vi "SpectralCoclustering.vi"(8 "error in":errorcluster) -> (0 "error out":errorcluster, 3 "out":refnum<class "SpectralCoclustering.lvclass">)   [LabVIEW 2020]
doc: "Spectral Co-Clustering algorithm (Dhillon, 2001).\n\n Clusters rows and columns of an array `X` to solve the relaxed\n normalized cut of the bipartite graph created from `X` as follows:\n the edge between row vertex `i` and column vertex `j` has weight\n `X[i, j]`.\n\n The resulting bicluster structure is block-diagonal, since each\n row and each column belongs to exactly one bicluster.\n\n Supports sparse matrices, as long as they are nonnegative.\n\n Read more in the :ref:`User Guide <spectral_coclustering>`.\n\n Parameters\n ----------\n n_clusters : int, default=3\n The number of biclusters to find.\n\n svd_method : {'randomized', 'arpack'}, default='randomized'\n Selects the algorithm for finding singular vectors. May be\n 'randomized' or 'arpack'. If 'randomized', use\n :func:`sklearn.utils.extmath.randomized_svd`, which may be faster\n for large matrices. If 'arpack', use\n :func:`scipy.sparse.linalg.svds`, which is more accurate, but\n possibly slower in some cases.\n\n n_svd_vecs : int, default=None\n Number of vectors to use in calculating the SVD. Corresponds\n to `ncv` when `svd_method=arpack` and `n_oversamples` when\n `svd_method` is 'randomized`.\n\n mini_batch : bool, default=False\n Whether to use mini-batch k-means, which is faster but may get\n different results.\n\n init : {'k-means++', 'random', or ndarray of shape (n_clusters, n_features), default='k-means++'\n Method for initialization of k-means algorithm; defaults to\n 'k-means++'.\n\n n_init : int, default=10\n Number of random initializations that are tried with the\n k-means algorithm.\n\n If mini-batch k-means is used, the best initialization is\n chosen and the algorithm runs once. Otherwise, the algorithm\n is run for each initialization and the best solution chosen.\n\n n_jobs : int, default=None\n The number of jobs to use for the computation. This works by breaking\n down the pairwise matrix into n_jobs even slices and computing them in\n parallel.\n\n ``None`` means 1 unless in a :obj:`joblib.parallel_backend` context.\n ``-1`` means using all processors. See :term:`Glossary <n_jobs>`\n for more details.\n\n .. deprecated:: 0.23\n ``n_jobs`` was deprecated in version 0.23 and will be removed in\n 1.0 (renaming of 0.25).\n\n random_state : int, RandomState instance, default=None\n Used for randomizing the singular value decomposition and the k-means\n initialization. Use an int to make the randomness deterministic.\n See :term:`Glossary <random_state>`.\n\n Attributes\n ----------\n rows_ : array-like of shape (n_row_clusters, n_rows)\n Results of the clustering. `rows[i, r]` is True if\n cluster `i` contains row `r`. Available only after calling ``fit``.\n\n columns_ : array-like of shape (n_column_clusters, n_columns)\n Results of the clustering, like `rows`.\n\n row_labels_ : array-like of shape (n_rows,)\n The bicluster label of each row.\n\n column_labels_ : array-like of shape (n_cols,)\n The bicluster label of each column.\n\n \nAvailable methods:\nGet Attributes\nGet Params\nSet Params"
uses:
  SpectralCoclustering.lvclass
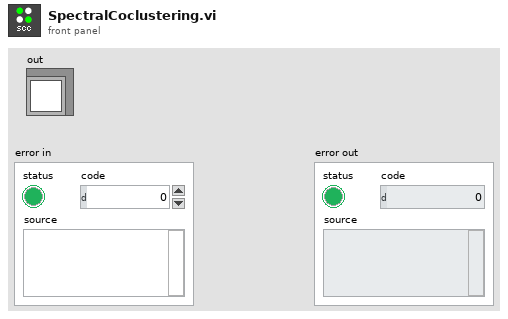
[diagram p1: front panel]
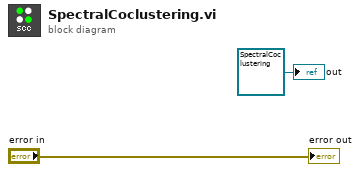
[diagram p0: block diagram]
diagram:
  "out" <- refnum<class "SpectralCoclustering.lvclass"> refnum ("model")
  "error out" <- "error in"
